vi "WLAN - TV - RW - UTIL - StringClusterToDataType.vi"(7 "TV Paramaters(String)":T4) -> (8 "WLAN Measurement Settings":T1={"OFDM Advanced Controls(11ag)"={"OFDM Auto Compute Acquisition Length Enabled"=0, "OFDM Maximum Symbols Used"=0, "OFDM Time Tracking Enabled"=0, "OFDM Channel Tracking Enabled"=0, "OFDM Amplitude Tracking Enabled"=1, "OFDM CFO Estimation Method"=0, "OFDM Phase Tracking Method"=0, "OFDM Header Detection Enabled"=0, "OFDM MAC FCS Check Enabled"=0, "#Avg"=10, "#Iterations"=10}, "DSSS Demod Parameters"={"DSSS Auto Compute Acquisition Length Enabled"=0, "DSSS Equalization Enabled"=0, "DSSS Header Detection Enabled"=0, "DSSS MAC FCS Check Enabled"=0, "DSSS Measurement Start Location"=0, "DSSS Phase Tracking Method"=0, "DSSS Maximum Chips Used"=0, "DSSS Reference Pulse Shaping Filter"=0, "DSSS Reference Pulse Shaping Filter Coefficient"=0.0, "# Avg"=1024, "# Iterations"=1024, "DSSS Power Ramp Enabled"=0}, "OFDM Advanced Controls (11n)"={"OFDM Auto Compute Acquisition Length Enabled"=0, "OFDM Maximum Symbols Used"=0, "OFDM Time Tracking Enabled"=0, "OFDM Channel Tracking Enabled"=0, "OFDM Amplitude Tracking Enabled"=1, "OFDM CFO Estimation Method"=0, "OFDM Phase Tracking Method"=0, "OFDM Header Detection Enabled"=0, "OFDM MAC FCS Check Enabled"=0, "#Avg"=10, "#Iterations"=10}, "OFDM Advanced Controls(11ac)"={"OFDM Auto Compute Acquisition Length Enabled"=0, "OFDM Maximum Symbols Used"=0, "OFDM Time Tracking Enabled"=1, "OFDM Channel Tracking Enabled"=0, "OFDM Amplitude Tracking Enabled"=0, "OFDM CFO Estimation Method"=0, "OFDM Phase Tracking Method"=0, "OFDM Header Detection Enabled"=0, "OFDM MAC FCS Check Enabled"=0, "#Avg"=10, "#Iterations"=10}} {"OFDM Advanced Controls(11ac)"."OFDM Phase Tracking Method" items=["Standard", "Instantaneous", "None", "Standard with Cubic Spline Fit"]; "OFDM Advanced Controls(11ac)"."OFDM CFO Estimation Method" items=["Preamble Only", "Preamble and Data"]; "OFDM Advanced Controls(11ac)"."OFDM Channel Tracking Enabled" items=["False", "True"]; "OFDM Advanced Controls(11ac)"."OFDM Amplitude Tracking Enabled" items=["False", "True"]; "OFDM Advanced Controls(11ac)"."OFDM Time Tracking Enabled" items=["True"=1, "False"=0]; "OFDM Advanced Controls(11ac)"."OFDM Auto Compute Acquisition Length Enabled" items=["False", "True"]; "OFDM Advanced Controls(11ac)"."OFDM MAC FCS Check Enabled" items=["False", "True"]; "OFDM Advanced Controls(11ac)"."OFDM Header Detection Enabled" items=["False", "True"]; "OFDM Advanced Controls (11n)"."OFDM Phase Tracking Method" items=["Standard", "Instantaneous", "None", "Standard with Cubic Spline Fit"]; "OFDM Advanced Controls (11n)"."OFDM CFO Estimation Method" items=["Preamble Only", "Preamble and Data"]; "OFDM Advanced Controls (11n)"."OFDM Channel Tracking Enabled" items=["False", "True"]; "OFDM Advanced Controls (11n)"."OFDM Amplitude Tracking Enabled" items=["False", "True"]; "OFDM Advanced Controls (11n)"."OFDM Time Tracking Enabled" items=["True"=1, "False"=0]; "OFDM Advanced Controls (11n)"."OFDM Auto Compute Acquisition Length Enabled" items=["False", "True"]; "OFDM Advanced Controls (11n)"."OFDM MAC FCS Check Enabled" items=["False", "True"]; "OFDM Advanced Controls (11n)"."OFDM Header Detection Enabled" items=["False", "True"]; "DSSS Demod Parameters"."DSSS Power Ramp Enabled" items=["False", "True"]; "DSSS Demod Parameters"."DSSS Auto Compute Acquisition Length Enabled" items=["False", "True"]; "DSSS Demod Parameters"."DSSS Phase Tracking Method" items=["Standard", "Instantaneous"]; "DSSS Demod Parameters"."DSSS Equalization Enabled" items=["False", "True"]; "DSSS Demod Parameters"."DSSS Reference Pulse Shaping Filter" items=["Rectangular", "Raised Cosine", "Root Raised Cosine", "Gaussian"]; "DSSS Demod Parameters"."DSSS MAC FCS Check Enabled" items=["False", "True"]; "DSSS Demod Parameters"."DSSS Header Detection Enabled" items=["False", "True"]; "OFDM Advanced Controls(11ag)"."OFDM Phase Tracking Method" items=["Standard", "Instantaneous", "None", "Standard with Cubic Spline Fit"]; "OFDM Advanced Controls(11ag)"."OFDM CFO Estimation Method" items=["Preamble Only", "Preamble and Data"]; "OFDM Advanced Controls(11ag)"."OFDM Channel Tracking Enabled" items=["False", "True"]; "OFDM Advanced Controls(11ag)"."OFDM Amplitude Tracking Enabled" items=["False", "True"]; "OFDM Advanced Controls(11ag)"."OFDM Time Tracking Enabled" items=["True"=1, "False"=0]; "OFDM Advanced Controls(11ag)"."OFDM Auto Compute Acquisition Length Enabled" items=["False", "True"]; "OFDM Advanced Controls(11ag)"."OFDM MAC FCS Check Enabled" items=["False", "True"]; "OFDM Advanced Controls(11ag)"."OFDM Header Detection Enabled" items=["False", "True"]})   [LabVIEW 2011]
uses:
  Includes/WLAN - TV - RW - INC - Tx_Measurement_Cluster(string).ctl
  Includes/WLAN - TV - RW - INC - Tx_Meas_Settings_OFDM_String.ctl
  Includes/WLAN - TV - RW - INC - Tx_Meas_Settings_DSSS_String.ctl
  Includes/WLAN - TV - RW - INC - Tx_Measurement_Cluster.ctl
  Includes/WLAN - TV - RW - INC - TV_OFDM Demod.ctl
  Includes/WLAN - TV - RW - INC - TV_DSSS Demod.ctl
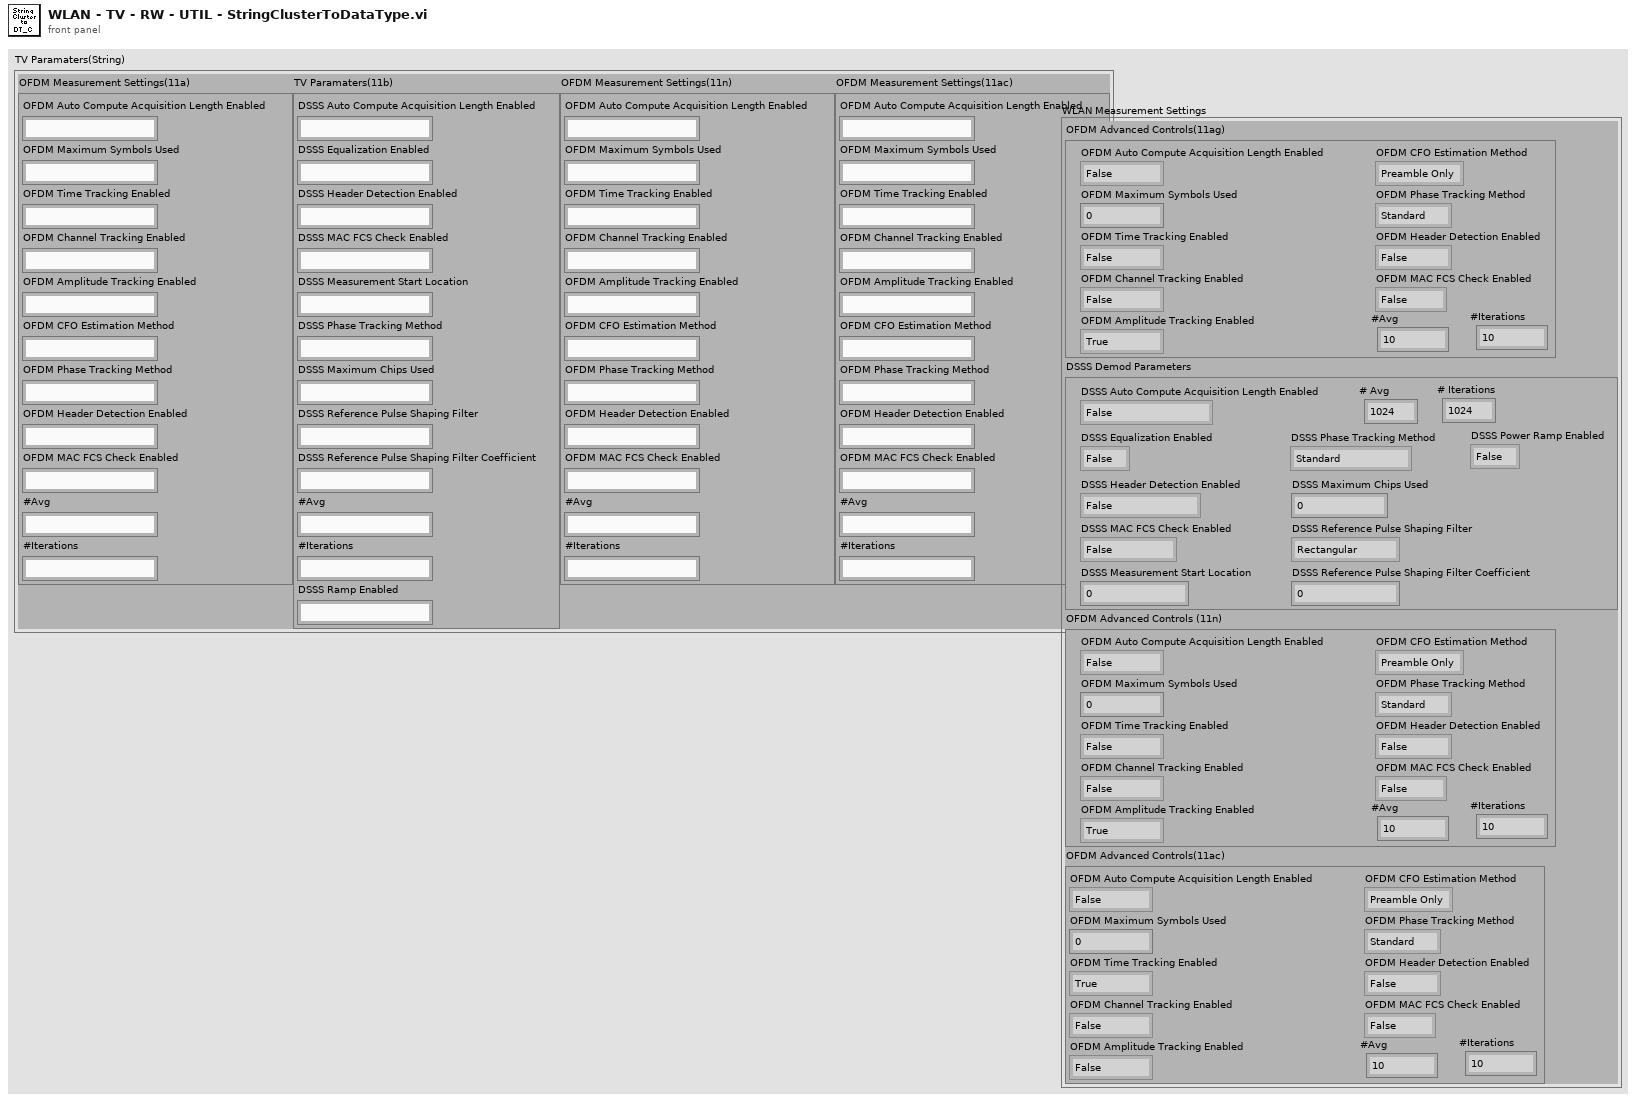
[diagram p1: front panel]
types:
  T1 = typedef "WLAN - TV - RW - INC - Tx_Measurement_Cluster.ctl" = cluster{"OFDM Advanced Controls(11ag)":T2, "DSSS Demod Parameters":T3, "OFDM Advanced Controls (11n)":T2, "OFDM Advanced Controls(11ac)":cluster{"OFDM Auto Compute Acquisition Length Enabled":i32, "OFDM Maximum Symbols Used":i32, "OFDM Time Tracking Enabled":i32, "OFDM Channel Tracking Enabled":i32, "OFDM Amplitude Tracking Enabled":i32, "OFDM CFO Estimation Method":i32, "OFDM Phase Tracking Method":i32, "OFDM Header Detection Enabled":i32, "OFDM MAC FCS Check Enabled":i32, "#Avg":i32, "#Iterations":i32}}
  T2 = typedef "WLAN - TV - RW - INC - TV_OFDM Demod.ctl" = cluster{"OFDM Auto Compute Acquisition Length Enabled":i32, "OFDM Maximum Symbols Used":i32, "OFDM Time Tracking Enabled":i32, "OFDM Channel Tracking Enabled":i32, "OFDM Amplitude Tracking Enabled":i32, "OFDM CFO Estimation Method":i32, "OFDM Phase Tracking Method":i32, "OFDM Header Detection Enabled":i32, "OFDM MAC FCS Check Enabled":i32, "#Avg":i32, "#Iterations":i32}
  T3 = typedef "WLAN - TV - RW - INC - TV_DSSS Demod.ctl" = cluster{"DSSS Auto Compute Acquisition Length Enabled":i32, "DSSS Equalization Enabled":i32, "DSSS Header Detection Enabled":i32, "DSSS MAC FCS Check Enabled":i32, "DSSS Measurement Start Location":i32, "DSSS Phase Tracking Method":i32, "DSSS Maximum Chips Used":i32, "DSSS Reference Pulse Shaping Filter":i32, "DSSS Reference Pulse Shaping Filter Coefficient":dbl, "# Avg":i32, "# Iterations":i32, "DSSS Power Ramp Enabled":i32}
  T4 = typedef "WLAN - TV - RW - INC - Tx_Measurement_Cluster(string).ctl" = cluster{"OFDM Measurement Settings(11a)":T5, "TV Paramaters(11b)":T6, "OFDM Measurement Settings(11n) ":T5, "OFDM Measurement Settings(11ac) ":T5}
  T5 = typedef "WLAN - TV - RW - INC - Tx_Meas_Settings_OFDM_String.ctl" = cluster{"OFDM Auto Compute Acquisition Length Enabled":string, "OFDM Maximum Symbols Used":string, "OFDM Time Tracking Enabled":string, "OFDM Channel Tracking Enabled":string, "OFDM Amplitude Tracking Enabled":string, "OFDM CFO Estimation Method":string, "OFDM Phase Tracking Method":string, "OFDM Header Detection Enabled":string, "OFDM MAC FCS Check Enabled":string, "#Avg":string, "#Iterations":string}
  T6 = typedef "WLAN - TV - RW - INC - Tx_Meas_Settings_DSSS_String.ctl" = cluster{"DSSS Auto Compute Acquisition Length Enabled":string, "DSSS Equalization Enabled":string, "DSSS Header Detection Enabled":string, "DSSS MAC FCS Check Enabled":string, "DSSS Measurement Start Location":string, "DSSS Phase Tracking Method":string, "DSSS Maximum Chips Used":string, "DSSS Reference Pulse Shaping Filter":string, "DSSS Reference Pulse Shaping Filter Coefficient":string, "#Avg":string, "#Iterations":string, "DSSS Ramp Enabled ":string}
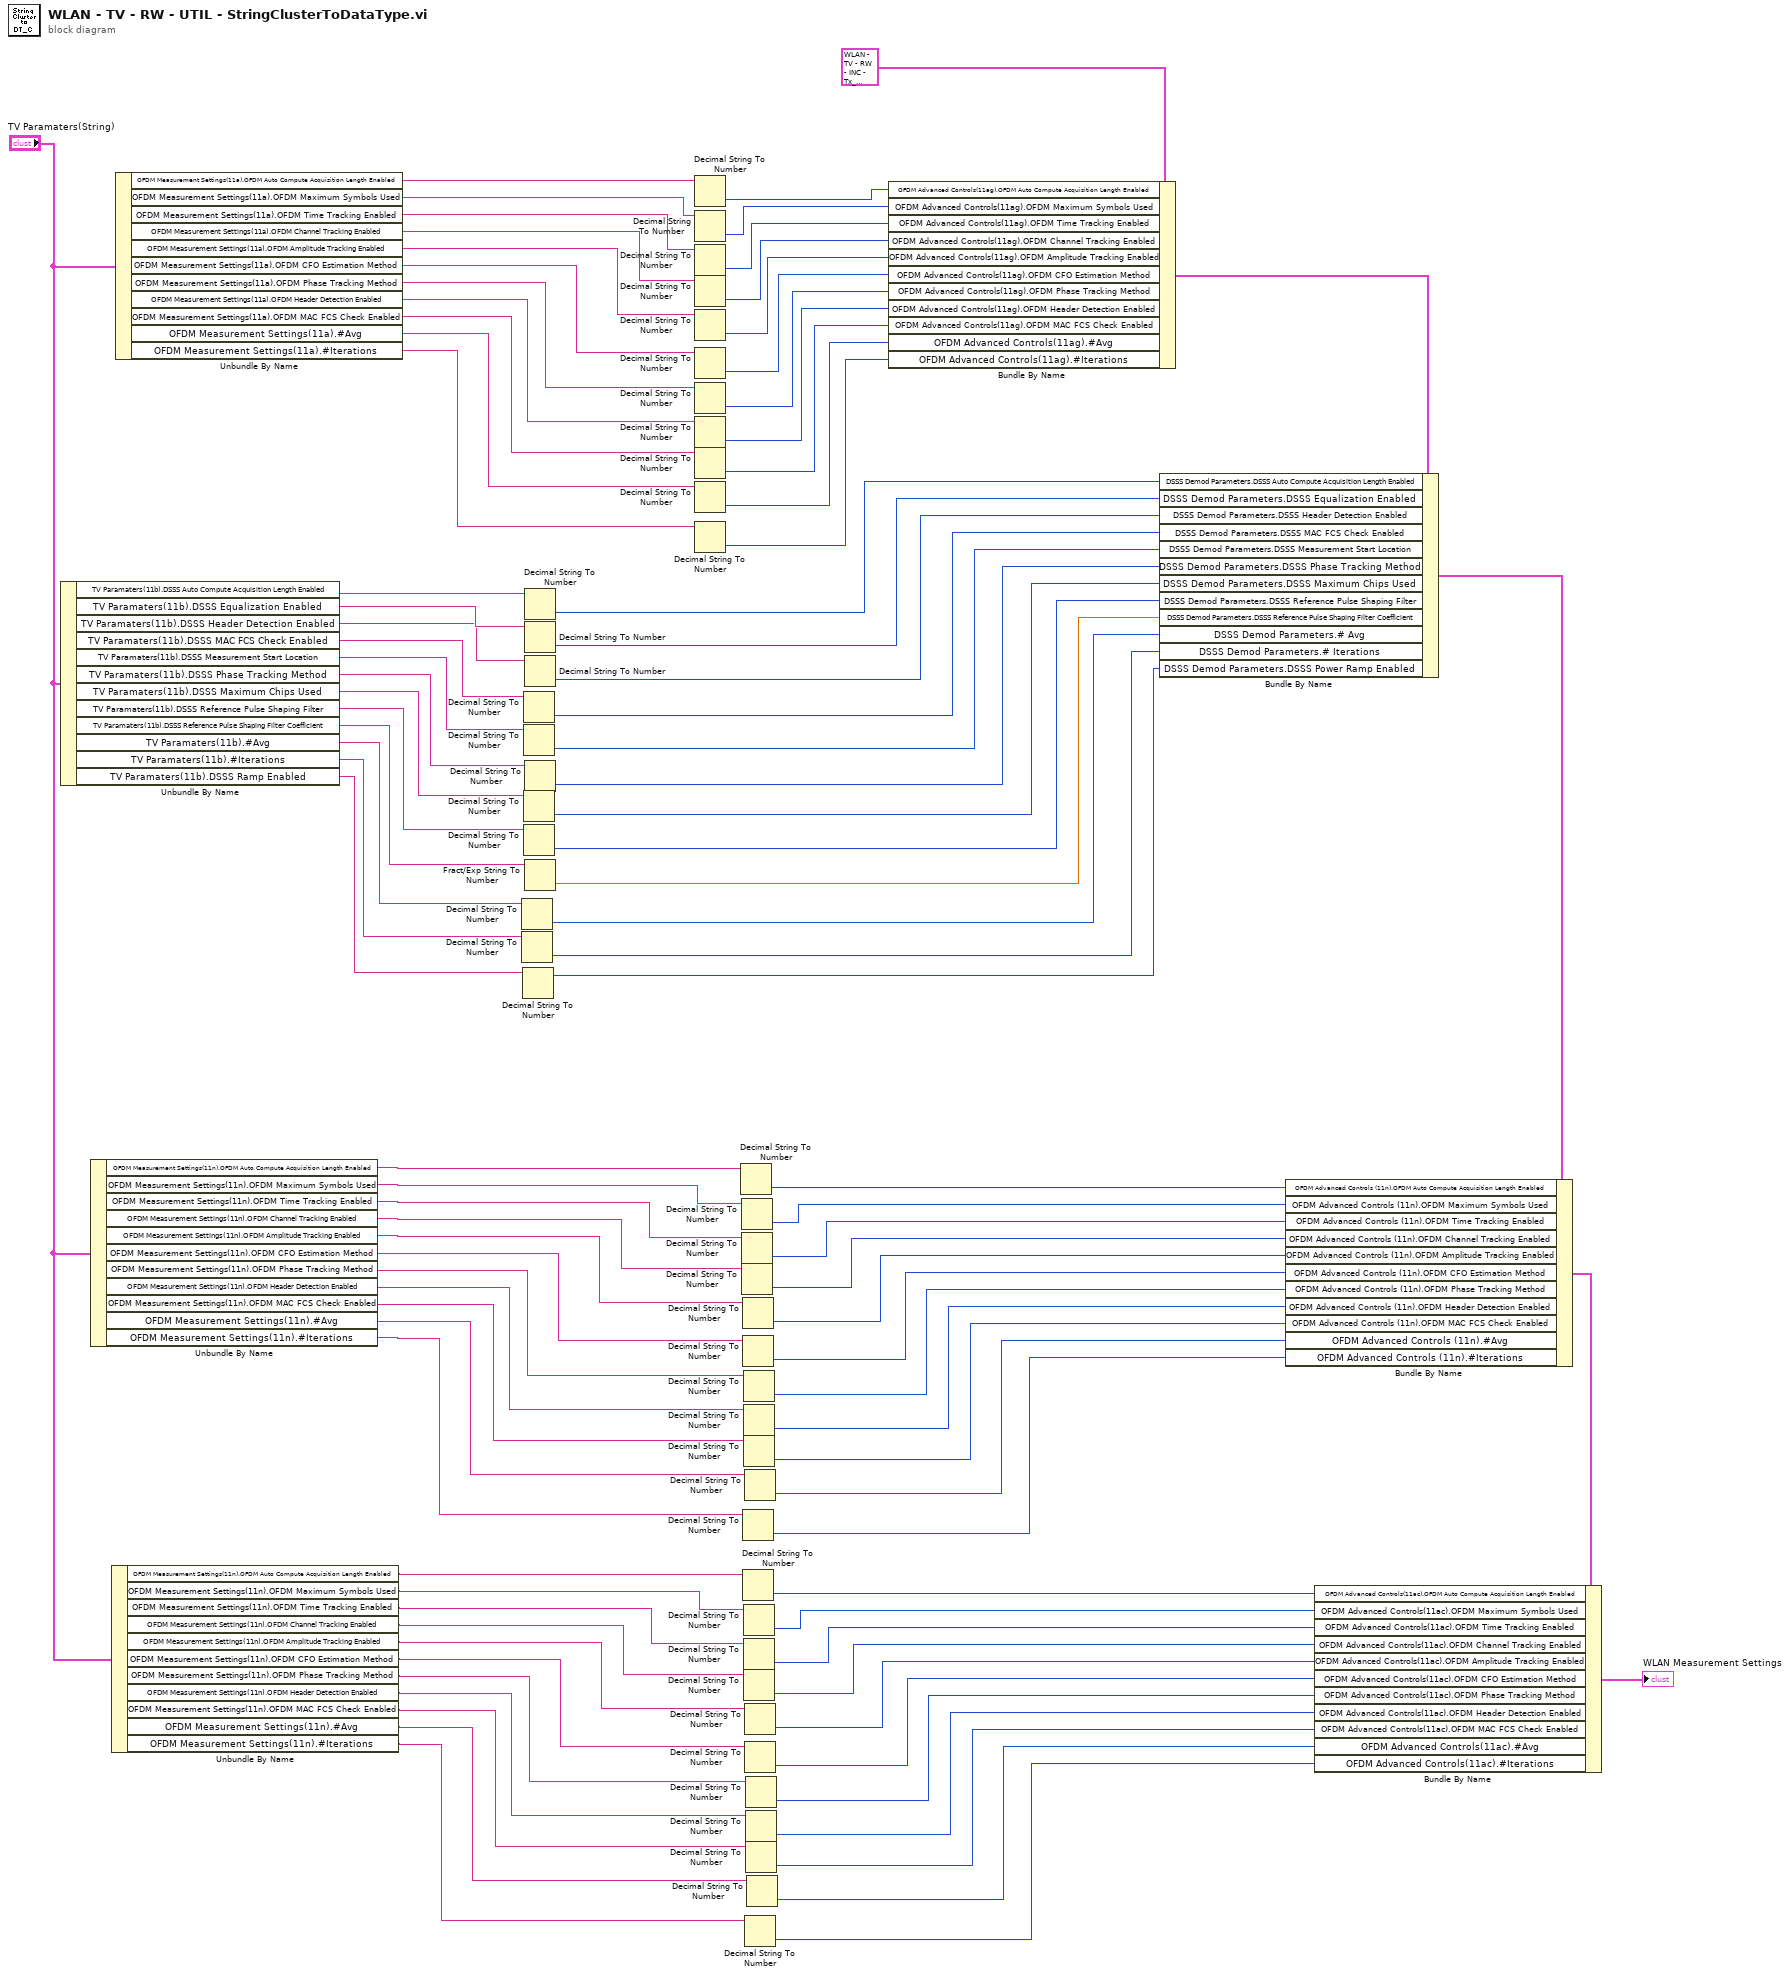
[diagram p0: block diagram]
diagram:
  n1 = Unbundle By Name("TV Paramaters(String)") -> ("TV Paramaters(11b).DSSS Auto Compute Acquisition Length Enabled"=w96:string, "TV Paramaters(11b).DSSS Equalization Enabled"=w95:string, "TV Paramaters(11b).DSSS Header Detection Enabled"=w94:string, "TV Paramaters(11b).DSSS MAC FCS Check Enabled"=w93:string, "TV Paramaters(11b).DSSS Measurement Start Location"=w92:string, "TV Paramaters(11b).DSSS Phase Tracking Method"=w41:string, "TV Paramaters(11b).DSSS Maximum Chips Used"=w91:string, "TV Paramaters(11b).DSSS Reference Pulse Shaping Filter"=w90:string, "TV Paramaters(11b).DSSS Reference Pulse Shaping Filter Coefficient"=w42:string, "TV Paramaters(11b).#Avg"=w89:string, "TV Paramaters(11b).#Iterations"=w88:string, "TV Paramaters(11b).DSSS Ramp Enabled"=w14:string)
  n2 = Unbundle By Name("TV Paramaters(String)") -> ("OFDM Measurement Settings(11n).OFDM Auto Compute Acquisition Length Enabled"=w11:string, "OFDM Measurement Settings(11n).OFDM Maximum Symbols Used"=w10:string, "OFDM Measurement Settings(11n).OFDM Time Tracking Enabled"=w9:string, "OFDM Measurement Settings(11n).OFDM Channel Tracking Enabled"=w8:string, "OFDM Measurement Settings(11n).OFDM Amplitude Tracking Enabled"=w7:string, "OFDM Measurement Settings(11n).OFDM CFO Estimation Method"=w6:string, "OFDM Measurement Settings(11n).OFDM Phase Tracking Method"=w5:string, "OFDM Measurement Settings(11n).OFDM Header Detection Enabled"=w4:string, "OFDM Measurement Settings(11n).OFDM MAC FCS Check Enabled"=w3:string, "OFDM Measurement Settings(11n).#Avg"=w2:string, "OFDM Measurement Settings(11n).#Iterations"=w1:string)
  n3 = Unbundle By Name("TV Paramaters(String)") -> ("OFDM Measurement Settings(11n).OFDM Auto Compute Acquisition Length Enabled"=w17:string, "OFDM Measurement Settings(11n).OFDM Maximum Symbols Used"=w18:string, "OFDM Measurement Settings(11n).OFDM Time Tracking Enabled"=w19:string, "OFDM Measurement Settings(11n).OFDM Channel Tracking Enabled"=w20:string, "OFDM Measurement Settings(11n).OFDM Amplitude Tracking Enabled"=w21:string, "OFDM Measurement Settings(11n).OFDM CFO Estimation Method"=w22:string, "OFDM Measurement Settings(11n).OFDM Phase Tracking Method"=w23:string, "OFDM Measurement Settings(11n).OFDM Header Detection Enabled"=w24:string, "OFDM Measurement Settings(11n).OFDM MAC FCS Check Enabled"=w25:string, "OFDM Measurement Settings(11n).#Avg"=w26:string, "OFDM Measurement Settings(11n).#Iterations"=w27:string)
  n4 = Unbundle By Name("TV Paramaters(String)") -> ("OFDM Measurement Settings(11a).OFDM Auto Compute Acquisition Length Enabled"=w87:string, "OFDM Measurement Settings(11a).OFDM Maximum Symbols Used"=w86:string, "OFDM Measurement Settings(11a).OFDM Time Tracking Enabled"=w85:string, "OFDM Measurement Settings(11a).OFDM Channel Tracking Enabled"=w84:string, "OFDM Measurement Settings(11a).OFDM Amplitude Tracking Enabled"=w83:string, "OFDM Measurement Settings(11a).OFDM CFO Estimation Method"=w82:string, "OFDM Measurement Settings(11a).OFDM Phase Tracking Method"=w81:string, "OFDM Measurement Settings(11a).OFDM Header Detection Enabled"=w80:string, "OFDM Measurement Settings(11a).OFDM MAC FCS Check Enabled"=w79:string, "OFDM Measurement Settings(11a).#Avg"=w78:string, "OFDM Measurement Settings(11a).#Iterations"=w77:string)
  n5 = Decimal String To Number(string=w89) -> (number=w62:i32)  [unwired: 2 in, 1 out]
  n6 = Decimal String To Number(string=w88) -> (number=w63:i32)  [unwired: 2 in, 1 out]
  n7 = Decimal String To Number(string=w14) -> (offset past number=w13:i32)  [unwired: 2 in, 1 out]
  n8 = Decimal String To Number(string=w93) -> (number=w58:i32)  [unwired: 2 in, 1 out]
  n9 = Decimal String To Number(string=w92) -> (number=w59:i32)  [unwired: 2 in, 1 out]
  n10 = Decimal String To Number(string=w91) -> (number=w60:i32)  [unwired: 2 in, 1 out]
  n11 = Decimal String To Number(string=w90) -> (number=w61:i32)  [unwired: 2 in, 1 out]
  n12 = Decimal String To Number(string=w96) -> (number=w55:i32)  [unwired: 2 in, 1 out]
  n13 = Decimal String To Number(string=w95) -> (number=w56:i32)  [unwired: 2 in, 1 out]
  n14 = Decimal String To Number(string=w94) -> (number=w57:i32)  [unwired: 2 in, 1 out]
  n15 = Decimal String To Number(string=w41) -> (number=w40:i32)  [unwired: 2 in, 1 out]
  n16 = Fract/Exp String To Number(string=w42) -> (number=w39:dbl)  [unwired: 3 in, 1 out]
  n17 = Decimal String To Number(string=w87) -> (number=w76:i32)  [unwired: 2 in, 1 out]
  n18 = Decimal String To Number(string=w86) -> (number=w74:i32)  [unwired: 2 in, 1 out]
  n19 = Decimal String To Number(string=w85) -> (number=w75:i32)  [unwired: 2 in, 1 out]
  n20 = Decimal String To Number(string=w84) -> (number=w72:i32)  [unwired: 2 in, 1 out]
  n21 = Decimal String To Number(string=w83) -> (number=w73:i32)  [unwired: 2 in, 1 out]
  n22 = Decimal String To Number(string=w82) -> (number=w71:i32)  [unwired: 2 in, 1 out]
  n23 = Decimal String To Number(string=w81) -> (number=w70:i32)  [unwired: 2 in, 1 out]
  n24 = Decimal String To Number(string=w80) -> (number=w69:i32)  [unwired: 2 in, 1 out]
  n25 = Decimal String To Number(string=w79) -> (number=w68:i32)  [unwired: 2 in, 1 out]
  n26 = Decimal String To Number(string=w78) -> (number=w67:i32)  [unwired: 2 in, 1 out]
  n27 = Decimal String To Number(string=w77) -> (number=w66:i32)  [unwired: 2 in, 1 out]
  n28 = Decimal String To Number(string=w11) -> (number=w53:i32)  [unwired: 2 in, 1 out]
  n29 = Decimal String To Number(string=w10) -> (number=w43:i32)  [unwired: 2 in, 1 out]
  n30 = Decimal String To Number(string=w9) -> (number=w44:i32)  [unwired: 2 in, 1 out]
  n31 = Decimal String To Number(string=w8) -> (number=w45:i32)  [unwired: 2 in, 1 out]
  n32 = Decimal String To Number(string=w7) -> (number=w46:i32)  [unwired: 2 in, 1 out]
  n33 = Decimal String To Number(string=w6) -> (number=w47:i32)  [unwired: 2 in, 1 out]
  n34 = Decimal String To Number(string=w1) -> (number=w52:i32)  [unwired: 2 in, 1 out]
  n35 = Decimal String To Number(string=w17) -> (number=w28:i32)  [unwired: 2 in, 1 out]
  n36 = Decimal String To Number(string=w5) -> (number=w48:i32)  [unwired: 2 in, 1 out]
  n37 = Decimal String To Number(string=w4) -> (number=w49:i32)  [unwired: 2 in, 1 out]
  n38 = Decimal String To Number(string=w3) -> (number=w50:i32)  [unwired: 2 in, 1 out]
  n39 = Decimal String To Number(string=w18) -> (number=w38:i32)  [unwired: 2 in, 1 out]
  n40 = Decimal String To Number(string=w19) -> (number=w37:i32)  [unwired: 2 in, 1 out]
  n41 = Decimal String To Number(string=w20) -> (number=w36:i32)  [unwired: 2 in, 1 out]
  n42 = Decimal String To Number(string=w2) -> (number=w51:i32)  [unwired: 2 in, 1 out]
  n43 = Decimal String To Number(string=w21) -> (number=w35:i32)  [unwired: 2 in, 1 out]
  n44 = Decimal String To Number(string=w22) -> (number=w34:i32)  [unwired: 2 in, 1 out]
  n45 = Decimal String To Number(string=w27) -> (number=w29:i32)  [unwired: 2 in, 1 out]
  n46 = Decimal String To Number(string=w23) -> (number=w33:i32)  [unwired: 2 in, 1 out]
  n47 = Decimal String To Number(string=w24) -> (number=w32:i32)  [unwired: 2 in, 1 out]
  n48 = Decimal String To Number(string=w25) -> (number=w31:i32)  [unwired: 2 in, 1 out]
  n49 = Decimal String To Number(string=w26) -> (number=w30:i32)  [unwired: 2 in, 1 out]
  n50 = Bundle By Name(cluster=T1 {"OFDM Advanced Controls(11ag)"={"OFDM Auto Compute Acquisition Length Enabled"=0, "OFDM Maximum Symbols Used"=0, "OFDM Time Tracking Enabled"=0, "OFDM Channel Tracking Enabled"=0, "OFDM Amplitude Tracking Enabled"=1, "OFDM CFO Estimation Method"=0, "OFDM Phase Tracking Method"=0, "OFDM Header Detection Enabled"=0, "OFDM MAC FCS Check Enabled"=0, "#Avg"=10, "#Iterations"=10}, "DSSS Demod Parameters"={"DSSS Auto Compute Acquisition Length Enabled"=0, "DSSS Equalization Enabled"=0, "DSSS Header Detection Enabled"=0, "DSSS MAC FCS Check Enabled"=0, "DSSS Measurement Start Location"=0, "DSSS Phase Tracking Method"=0, "DSSS Maximum Chips Used"=0, "DSSS Reference Pulse Shaping Filter"=0, "DSSS Reference Pulse Shaping Filter Coefficient"=0.0, "# Avg"=1024, "# Iterations"=1024, "DSSS Power Ramp Enabled"=0}, "OFDM Advanced Controls (11n)"={"OFDM Auto Compute Acquisition Length Enabled"=0, "OFDM Maximum Symbols Used"=0, "OFDM Time Tracking Enabled"=0, "OFDM Channel Tracking Enabled"=0, "OFDM Amplitude Tracking Enabled"=1, "OFDM CFO Estimation Method"=0, "OFDM Phase Tracking Method"=0, "OFDM Header Detection Enabled"=0, "OFDM MAC FCS Check Enabled"=0, "#Avg"=10, "#Iterations"=10}, "OFDM Advanced Controls(11ac)"={"OFDM Auto Compute Acquisition Length Enabled"=0, "OFDM Maximum Symbols Used"=0, "OFDM Time Tracking Enabled"=0, "OFDM Channel Tracking Enabled"=0, "OFDM Amplitude Tracking Enabled"=0, "OFDM CFO Estimation Method"=0, "OFDM Phase Tracking Method"=0, "OFDM Header Detection Enabled"=0, "OFDM MAC FCS Check Enabled"=0, "#Avg"=0, "#Iterations"=0}} ("WLAN Measurement Settings"), "OFDM Advanced Controls(11ag).OFDM Auto Compute Acquisition Length Enabled"=w76, "OFDM Advanced Controls(11ag).OFDM Maximum Symbols Used"=w74, "OFDM Advanced Controls(11ag).OFDM Time Tracking Enabled"=w75, "OFDM Advanced Controls(11ag).OFDM Channel Tracking Enabled"=w72, "OFDM Advanced Controls(11ag).OFDM Amplitude Tracking Enabled"=w73, "OFDM Advanced Controls(11ag).OFDM CFO Estimation Method"=w71, "OFDM Advanced Controls(11ag).OFDM Phase Tracking Method"=w70, "OFDM Advanced Controls(11ag).OFDM Header Detection Enabled"=w69, "OFDM Advanced Controls(11ag).OFDM MAC FCS Check Enabled"=w68, "OFDM Advanced Controls(11ag).#Avg"=w67, "OFDM Advanced Controls(11ag).#Iterations"=w66) -> (w64:T1)
  n51 = Bundle By Name(cluster=w64, "DSSS Demod Parameters.DSSS Auto Compute Acquisition Length Enabled"=w55, "DSSS Demod Parameters.DSSS Equalization Enabled"=w56, "DSSS Demod Parameters.DSSS Header Detection Enabled"=w57, "DSSS Demod Parameters.DSSS MAC FCS Check Enabled"=w58, "DSSS Demod Parameters.DSSS Measurement Start Location"=w59, "DSSS Demod Parameters.DSSS Phase Tracking Method"=w40, "DSSS Demod Parameters.DSSS Maximum Chips Used"=w60, "DSSS Demod Parameters.DSSS Reference Pulse Shaping Filter"=w61, "DSSS Demod Parameters.DSSS Reference Pulse Shaping Filter Coefficient"=w39, "DSSS Demod Parameters.# Avg"=w62, "DSSS Demod Parameters.# Iterations"=w63, "DSSS Demod Parameters.DSSS Power Ramp Enabled"=w13) -> (w54:T1)
  n52 = Bundle By Name(cluster=w54, "OFDM Advanced Controls (11n).OFDM Auto Compute Acquisition Length Enabled"=w53, "OFDM Advanced Controls (11n).OFDM Maximum Symbols Used"=w43, "OFDM Advanced Controls (11n).OFDM Time Tracking Enabled"=w44, "OFDM Advanced Controls (11n).OFDM Channel Tracking Enabled"=w45, "OFDM Advanced Controls (11n).OFDM Amplitude Tracking Enabled"=w46, "OFDM Advanced Controls (11n).OFDM CFO Estimation Method"=w47, "OFDM Advanced Controls (11n).OFDM Phase Tracking Method"=w48, "OFDM Advanced Controls (11n).OFDM Header Detection Enabled"=w49, "OFDM Advanced Controls (11n).OFDM MAC FCS Check Enabled"=w50, "OFDM Advanced Controls (11n).#Avg"=w51, "OFDM Advanced Controls (11n).#Iterations"=w52) -> (w16:T1)
  n53 = Bundle By Name(cluster=w16, "OFDM Advanced Controls(11ac).OFDM Auto Compute Acquisition Length Enabled"=w28, "OFDM Advanced Controls(11ac).OFDM Maximum Symbols Used"=w38, "OFDM Advanced Controls(11ac).OFDM Time Tracking Enabled"=w37, "OFDM Advanced Controls(11ac).OFDM Channel Tracking Enabled"=w36, "OFDM Advanced Controls(11ac).OFDM Amplitude Tracking Enabled"=w35, "OFDM Advanced Controls(11ac).OFDM CFO Estimation Method"=w34, "OFDM Advanced Controls(11ac).OFDM Phase Tracking Method"=w33, "OFDM Advanced Controls(11ac).OFDM Header Detection Enabled"=w32, "OFDM Advanced Controls(11ac).OFDM MAC FCS Check Enabled"=w31, "OFDM Advanced Controls(11ac).#Avg"=w30, "OFDM Advanced Controls(11ac).#Iterations"=w29) -> (→"WLAN Measurement Settings":T1)
